vi "Inverse_MpembaDW.vi"(0 "Xpos":sgl, 1 "ktrap*mob":sgl, 5 "Xm":sgl, 9 "Eb":sgl, 11 "dE":sgl, 12 "Fmax":sgl, 13 "Xmax":sgl, 14 "Xmin":sgl=-1.0) -> (6 "DWvolt":sgl)   [LabVIEW 2019]
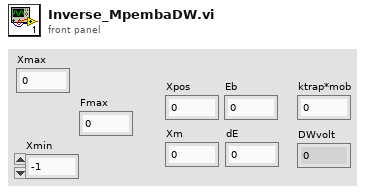
[diagram p1: front panel]
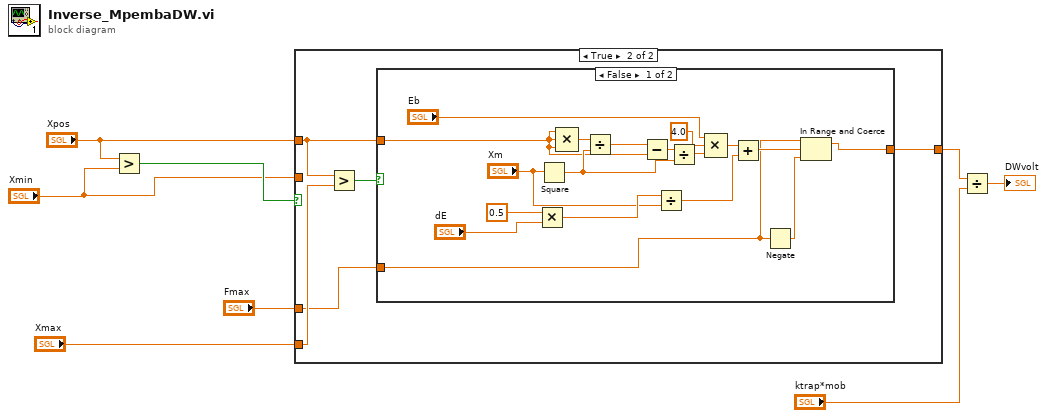
[diagram p0: block diagram]
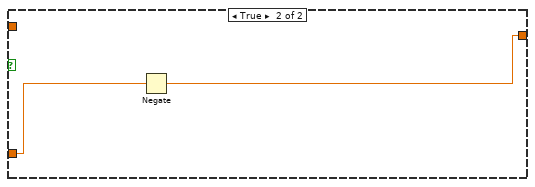
[diagram p3: hidden frame]
diagram:
  n1 = Greater?(x="Xpos", y="Xmin") -> (0:w6:bool)
  n2 = case shown="True" w6 {
    tunnel: "Xpos" -> [_ w13]
    tunnel: [w9 w14] -> w4
    tunnel: "Xmax" -> [_ w11]
    tunnel: "Fmax" -> [w9 w10]
    tunnel: "Xmin" -> [_ _]
    frame False {
    }
    frame True {
      n3 = Greater?(x=w13, y=w11) -> (0:w12:bool)
      n4 = case shown="False" w12 {
        tunnel: w13 -> [w19 _]
        tunnel: [w17 w33] -> w14
        tunnel: w10 -> [w15 w34]
        frame False {
          n5 = Multiply(x=sgl 0.5 ("y"), y="dE") -> (x*y=w26:sgl)
          n6 = Square(x="Xm") -> (x^2=w28:sgl)
          n7 = Compound Arithmetic op=MULTIPLY(w19, w19, w19) -> (w30:sgl)
          n8 = Divide(x=w30, y=w28) -> (x/y=w20:sgl)
          n9 = Subtract(x=w20, y=w19) -> (x-y=w29:sgl)
          n10 = Divide(x=w26, y="Xm") -> (x/y=w23:sgl)
          n11 = Divide(x=w29, y=w28) -> (x/y=w32:sgl)
          n12 = Compound Arithmetic op=MULTIPLY("Eb", sgl 4.0 ("value"), w32) -> (w24:sgl)
          n13 = Add(x=w24, y=w23) -> (x+y=w18:sgl)
          n14 = Negate(x=w15) -> (-x=w16:sgl)
          n15 = In Range and Coerce(upper limit=w15, x=w18, lower limit=w16) -> (coerced(x)=w17:sgl)  [unwired: 1 out]
        }
        frame True {
          n16 = Negate(x=w34) -> (-x=w33:sgl)
        }
      }
    }
  }
  n17 = Divide(x=w4, y="ktrap*mob") -> (x/y=→"DWvolt":sgl)
